vi "InvalidConfiguration.vi"(8 "error in (no error)":errorcluster, 10 "description":string, 11 "Qbus in":refnum<class "Qbus.lvclass">) -> (0 "error out":errorcluster, 3 "Qbus out":refnum<class "Qbus.lvclass">)   [LabVIEW 2017, in "Qbus.lvclass"]
uses:
  <vilib>/addons/Qbus/Qbus.lvclass
  <vilib>/addons/Qbus/Qbus.lvclass/Qbus.ctl
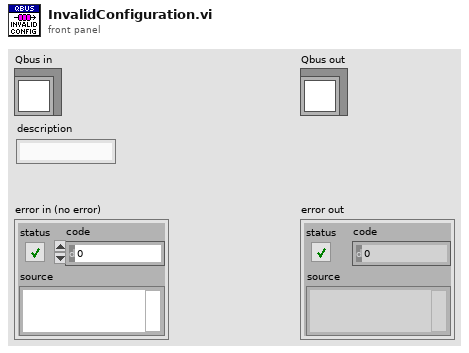
[diagram p1: front panel]
types:
  T1 = typedef "Qbus.lvclass/data.ctl" = cluster{"Queues":variant, "Subscriptions":variant, "MasterQ":string}
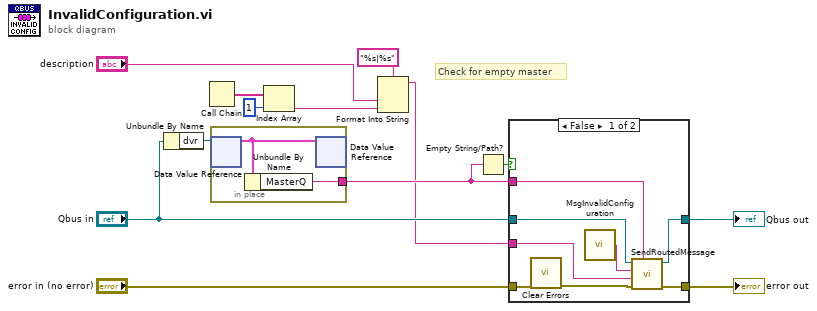
[diagram p0: block diagram]
diagram:
  # "Check for empty master"
  n1 = Unbundle By Name("Qbus in") -> ("dvr"=w6:refnum<data-value>)
  n2 = Call Chain() -> (call chain=w8:string[])
  n3 = in-place {
    in-place-border: [w14] -> w5
    n4 = in-place-dvr #1(w6) -> (w15:T1)  [unwired: 1 out]
    n5 = Unbundle By Name(w15) -> ("MasterQ"=w14:string)
    n6 = in-place-dvr #1(w15) -> ()  [unwired: 2 out]
  }
  n7 = Index Array(array=w8, index=1) -> (element=w1:string)
  n8 = Format Into String(format string="%s|%s", "description", w1) -> (resulting string=w2:string)  [unwired: 2 in, 1 out]
  n9 = Empty String/Path?(string/path=w5) -> (empty?=w4:bool)
  n10 = case shown="False" w4 {
    tunnel: "error in (no error)" -> [w18 w24]
    tunnel: [w23 w25] -> w10
    tunnel: [w22 w24] -> w9
    tunnel: w2 -> [w21 _]
    tunnel: "Qbus in" -> [w20 w25]
    tunnel: w5 -> [w19 _]
    frame False {
      n11 = call <vilib>:"Clear Errors.vi"("error in (no error)"=w18) -> ("error out"=w17:errorcluster)  [unwired: 5 in, 1 out]
      n12 = call <vilib>:"MsgInvalidConfiguration.vi"() -> ("message name"=w16:string)  [unwired: 5 in]
      n13 = call <vilib>:"SendRoutedMessage.vi"("listener process"=w19, "error in (no error)"=w17, "message value"=w21, "message name"=w16, "Qbus in"=w20) -> ("error in (no error)"=w22:errorcluster, "Qbus out"=w23:refnum<class "Qbus.lvclass">)  [unwired: 5 in]
    }
    frame True {
    }
  }
  "error out" <- w9
  "Qbus out" <- w10
